vi "Close Transport.vi"(8 "error in (no error)":errorcluster, 11 "StreamToDiskTransport":refnum<class "StreamToDiskTransport.lvclass">) -> (0 "error out":errorcluster)   [LabVIEW 2015, in "Transport.lvlib" / "StreamToDiskTransport.lvclass"]
uses:
  StreamToDiskTransport.lvclass
  StreamToDiskTransport.lvclass/StreamToDiskTransport.ctl
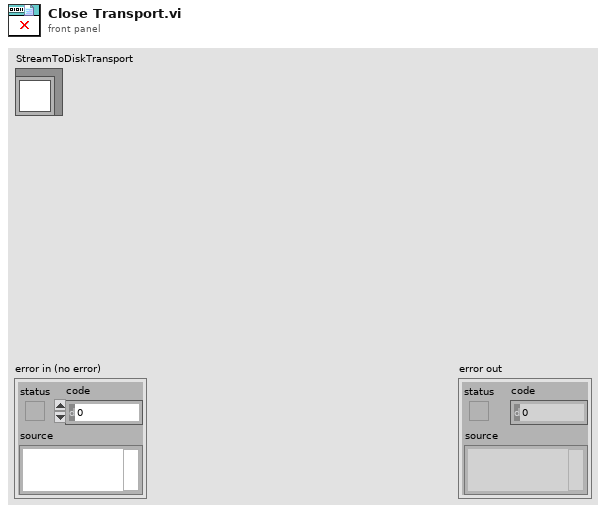
[diagram p1: front panel]
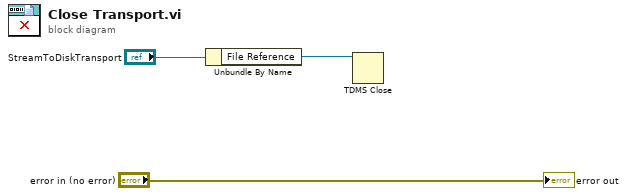
[diagram p0: block diagram]
diagram:
  n1 = Unbundle By Name("StreamToDiskTransport") -> ("File Reference"=w1:refnum<k34>)
  n2 = TDMS Close(11:w1) -> ()  [unwired: 1 in, 2 out]
  "error out" <- "error in (no error)"
